vi "TestTransformTokenizer.vi"(8 "error in (no error)":errorcluster) -> (0 "error out":errorcluster)   [LabVIEW 2019]
uses:
  TransformTokenizer/TransformTokenizer.lvclass
  TransformTokenizer/TransformTokenizer.lvclass/TransformTokenizer.ctl
  <vilib>/addons/_JKI Toolkits/Caraya/classes/Assert/Assert Equal Value_Variant.vi
  <vilib>/addons/_JKI Toolkits/Caraya/classes/Test/Test.lvclass
  <vilib>/addons/_JKI Toolkits/Caraya/classes/Assert/Assert.lvclass
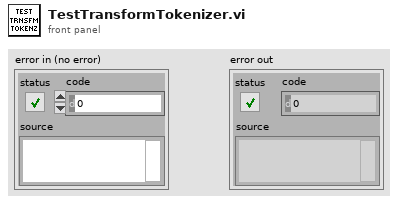
[diagram p1: front panel]
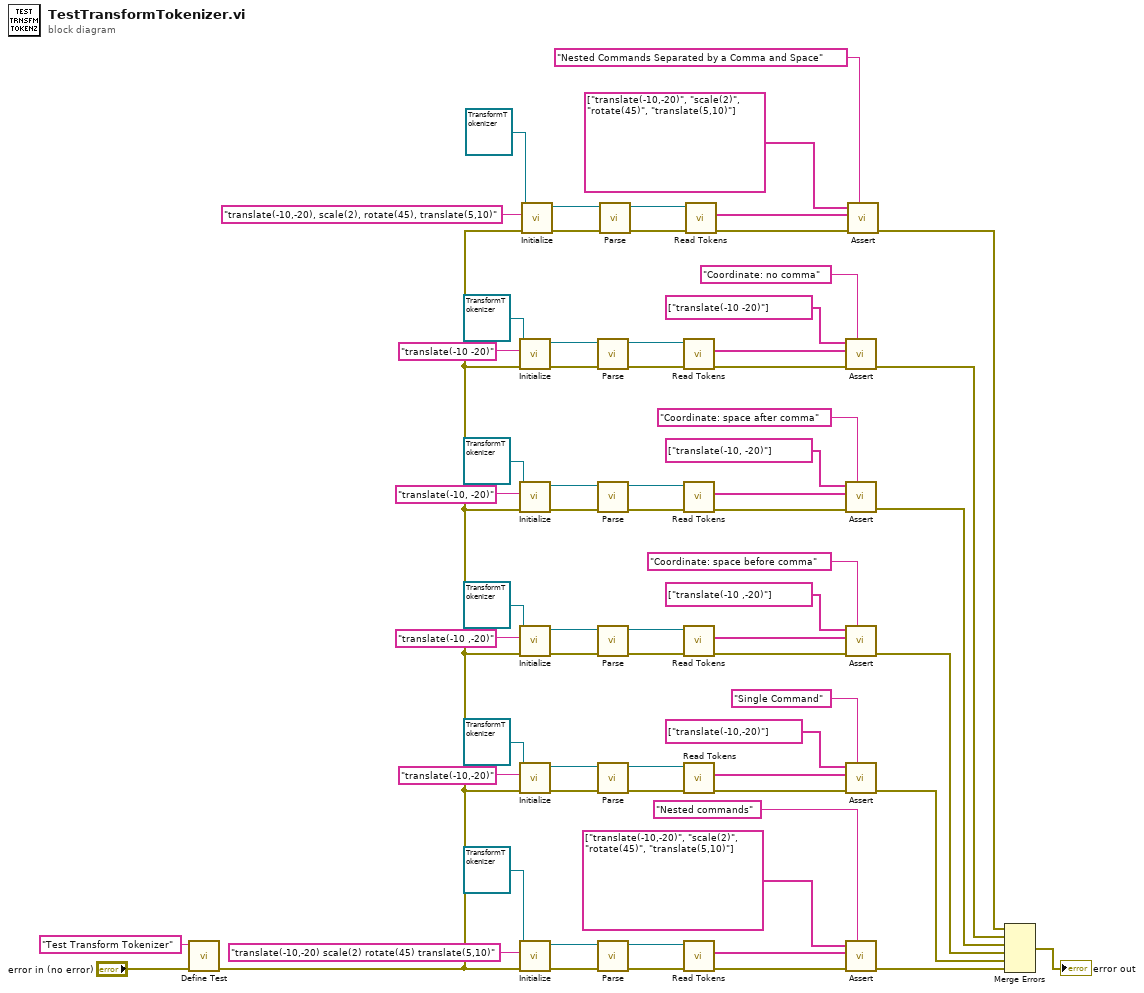
[diagram p0: block diagram]
diagram:
  n1 = call <vilib>:"Define Test.vi"("error in (no error)"="error in (no error)", "Label (VI Title)"="Test Transform Tokenizer") -> ("error out"=w4:errorcluster)  [unwired: 8 in, 1 out]
  n2 = call "Initialize.vi"("error in (no error)"=w4, "Transform Attribute String"="translate(-10 -20)", "TransformTokenizer in"=refnum<class "TransformTokenizer.lvclass"> refnum) -> ("error out"=w14:errorcluster, "TransformTokenizer out"=w15:refnum<class "TransformTokenizer.lvclass">)  [unwired: 7 in]
  n3 = call "Initialize.vi"("error in (no error)"=w4, "Transform Attribute String"="translate(-10, -20)", "TransformTokenizer in"=refnum<class "TransformTokenizer.lvclass"> refnum) -> ("error out"=w34:errorcluster, "TransformTokenizer out"=w33:refnum<class "TransformTokenizer.lvclass">)  [unwired: 7 in]
  n4 = call "Initialize.vi"("error in (no error)"=w4, "Transform Attribute String"="translate(-10 ,-20)", "TransformTokenizer in"=refnum<class "TransformTokenizer.lvclass"> refnum) -> ("error out"=w36:errorcluster, "TransformTokenizer out"=w37:refnum<class "TransformTokenizer.lvclass">)  [unwired: 7 in]
  n5 = call "Initialize.vi"("error in (no error)"=w4, "Transform Attribute String"="translate(-10,-20)", "TransformTokenizer in"=refnum<class "TransformTokenizer.lvclass"> refnum) -> ("error out"=w56:errorcluster, "TransformTokenizer out"=w55:refnum<class "TransformTokenizer.lvclass">)  [unwired: 7 in]
  n6 = call "Initialize.vi"("error in (no error)"=w4, "Transform Attribute String"="translate(-10,-20) scale(2) rotate(45) translate(5,10)", "TransformTokenizer in"=refnum<class "TransformTokenizer.lvclass"> refnum) -> ("error out"=w63:errorcluster, "TransformTokenizer out"=w64:refnum<class "TransformTokenizer.lvclass">)  [unwired: 7 in]
  n7 = call "Initialize.vi"("error in (no error)"=w4, "Transform Attribute String"="translate(-10,-20), scale(2), rotate(45), translate(5,10)", "TransformTokenizer in"=refnum<class "TransformTokenizer.lvclass"> refnum) -> ("error out"=w9:errorcluster, "TransformTokenizer out"=w10:refnum<class "TransformTokenizer.lvclass">)  [unwired: 7 in]
  n8 = call "Parse.vi"("error in (no error)"=w14, "TransformTokenizer in"=w15) -> ("error out"=w16:errorcluster, "TransformTokenizer out"=w17:refnum<class "TransformTokenizer.lvclass">)  [unwired: 8 in]
  n9 = call "Parse.vi"("error in (no error)"=w34, "TransformTokenizer in"=w33) -> ("error out"=w32:errorcluster, "TransformTokenizer out"=w31:refnum<class "TransformTokenizer.lvclass">)  [unwired: 8 in]
  n10 = call "Parse.vi"("error in (no error)"=w36, "TransformTokenizer in"=w37) -> ("error out"=w38:errorcluster, "TransformTokenizer out"=w39:refnum<class "TransformTokenizer.lvclass">)  [unwired: 8 in]
  n11 = call "Parse.vi"("error in (no error)"=w56, "TransformTokenizer in"=w55) -> ("error out"=w54:errorcluster, "TransformTokenizer out"=w53:refnum<class "TransformTokenizer.lvclass">)  [unwired: 8 in]
  n12 = call "Parse.vi"("error in (no error)"=w63, "TransformTokenizer in"=w64) -> ("error out"=w65:errorcluster, "TransformTokenizer out"=w66:refnum<class "TransformTokenizer.lvclass">)  [unwired: 8 in]
  n13 = call "Parse.vi"("error in (no error)"=w9, "TransformTokenizer in"=w10) -> ("error out"=w11:errorcluster, "TransformTokenizer out"=w12:refnum<class "TransformTokenizer.lvclass">)  [unwired: 8 in]
  n14 = call "Read Tokens.vi"("error in (no error)"=w16, "TransformTokenizer in"=w17) -> ("error out"=w20:errorcluster, "Transforms"=w21:string[])  [unwired: 7 in, 1 out]
  n15 = call "Read Tokens.vi"("error in (no error)"=w32, "TransformTokenizer in"=w31) -> ("error out"=w28:errorcluster, "Transforms"=w27:string[])  [unwired: 7 in, 1 out]
  n16 = call "Read Tokens.vi"("error in (no error)"=w38, "TransformTokenizer in"=w39) -> ("error out"=w42:errorcluster, "Transforms"=w43:string[])  [unwired: 7 in, 1 out]
  n17 = call "Read Tokens.vi"("error in (no error)"=w54, "TransformTokenizer in"=w53) -> ("error out"=w50:errorcluster, "Transforms"=w48:string[])  [unwired: 7 in, 1 out]
  n18 = call "Read Tokens.vi"("error in (no error)"=w65, "TransformTokenizer in"=w66) -> ("error out"=w67:errorcluster, "Transforms"=w60:string[])  [unwired: 7 in, 1 out]
  n19 = call "Read Tokens.vi"("error in (no error)"=w11, "TransformTokenizer in"=w12) -> ("error out"=w13:errorcluster, "Transforms"=w7:string[])  [unwired: 7 in, 1 out]
  n20 = call-poly <vilib>:"Assert.vi"("Label"="Coordinate: no comma", "error in (no error)"=w20, "Y"=w21, "X"=string[] ["translate(-10 -20)"] ("Transforms")) -> ("error out"=w1:errorcluster)  [unwired: 6 in, 1 out]
  n21 = call-poly <vilib>:"Assert.vi"("Label"="Coordinate: space after comma", "error in (no error)"=w28, "Y"=w27, "X"=string[] ["translate(-10, -20)"] ("Transforms")) -> ("error out"=w24:errorcluster)  [unwired: 6 in, 1 out]
  n22 = call-poly <vilib>:"Assert.vi"("Label"="Coordinate: space before comma", "error in (no error)"=w42, "Y"=w43, "X"=string[] ["translate(-10 ,-20)"] ("Transforms")) -> ("error out"=w35:errorcluster)  [unwired: 6 in, 1 out]
  n23 = call-poly <vilib>:"Assert.vi"("Label"="Single Command", "error in (no error)"=w50, "Y"=w48, "X"=string[] ["translate(-10,-20)"] ("Transforms")) -> ("error out"=w49:errorcluster)  [unwired: 6 in, 1 out]
  n24 = call-poly <vilib>:"Assert.vi"("Label"="Nested commands", "error in (no error)"=w67, "Y"=w60, "X"=string[] ["translate(-10,-20)", "scale(2)", "rotate(45)", "translate(5,10)"] ("Transforms")) -> ("error out"=w61:errorcluster)  [unwired: 6 in, 1 out]
  n25 = call-poly <vilib>:"Assert.vi"("Label"="Nested Commands Separated by a Comma and Space", "error in (no error)"=w13, "Y"=w7, "X"=string[] ["translate(-10,-20)", "scale(2)", "rotate(45)", "translate(5,10)"] ("Transforms")) -> ("error out"=w2:errorcluster)  [unwired: 6 in, 1 out]
  n26 = Merge Errors(w2, w1, w24, w35, w49, w61) -> (→"error out":errorcluster)
